vi "Safety Sensor Alarm.vi"(10 "Safety":bool, 11 "Reset":bool) -> ()   [LabVIEW 2015]
uses:
  Galobal variable_TI.vi
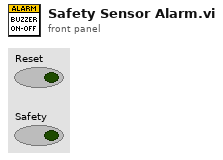
[diagram p1: front panel]
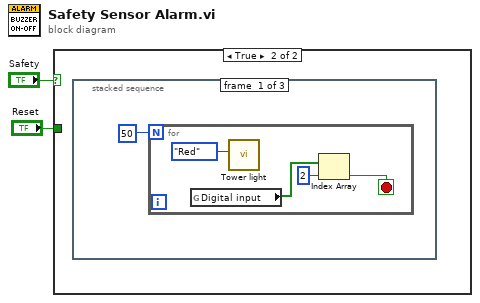
[diagram p0: block diagram]
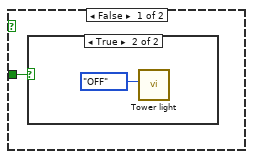
[diagram p2: hidden frame]
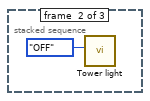
[diagram p4: hidden frame]
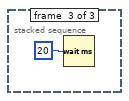
[diagram p5: hidden frame]
diagram:
  n1 = case shown="True" "Safety" {
    tunnel: "Reset" -> [w3 _]
    frame False {
      n2 = case shown="True" w3 {
        frame False {
        }
        frame True {
          n3 = call "Tower light.vi"("Enum"=enum16{"Green", "Red", "Yellow", "OFF"}."OFF") -> ()  [unwired: 11 in]
        }
      }
    }
    frame True {
      n4 = stacked-sequence {
        frame #0 {
          n5 = for {
            N: 50 -> [_]
            stop <- w6 stop-if-true
            n6 = global read "Galobal variable_TI.vi" "Digital input"() -> (w8:bool[])
            n7 = call "Tower light.vi"("Enum"=enum16{"Green", "Red", "Yellow", "OFF"}."Red") -> ()  [unwired: 11 in]
            n8 = Index Array(array=w8, index=2) -> (element=w6:bool)
          }
        }
        frame #1 {
          n9 = call "Tower light.vi"("Enum"=enum16{"Green", "Red", "Yellow", "OFF"}."OFF") -> ()  [unwired: 11 in]
        }
        frame #2 {
          n10 = Wait (ms)(milliseconds to wait=u32 20) -> ()  [unwired: 1 out]
        }
      }
    }
  }
